vi "Read VI For Changes.vi"(8 "error in (no error)":errorcluster, 10 "Current VI Data":T1, 11 "VI Refnum":refnum<vi>) -> (0 "error out":errorcluster, 1 "ChangeInData?":bool, 2 "Updated VI Data":T1)   [LabVIEW 2014, in "SmartPalette.lvlib"]
uses:
  SmartPalette.lvlib
  Controls/VI - DataStorage.ctl
  Controls/GObjectDetail.ctl
  <vilib>/Utility/traverseref.llb/TRef TravTarget.ctl
  <vilib>/Utility/traverseref.llb/VI Scripting - Traverse.lvlib
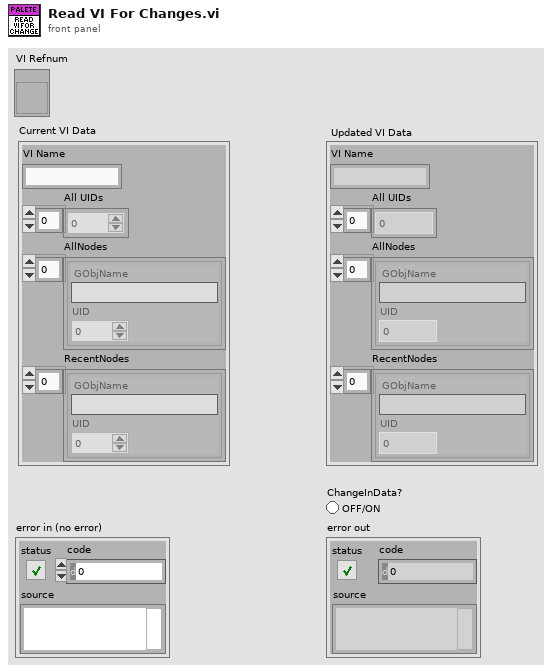
[diagram p1: front panel]
types:
  T1 = typedef "SmartPalette.lvlib/VI - DataStorage.ctl" = cluster{"VI Name":string, "All UIDs":i32[], "AllNodes":T2[], "RecentNodes":T2[]}
  T2 = typedef "SmartPalette.lvlib/GObjectDetail.ctl" = cluster{"GObjName":string, "UID":i32}
  T3 = typedef "TRef TravTarget.ctl" = enum16{"FP", "BD", "Other"}
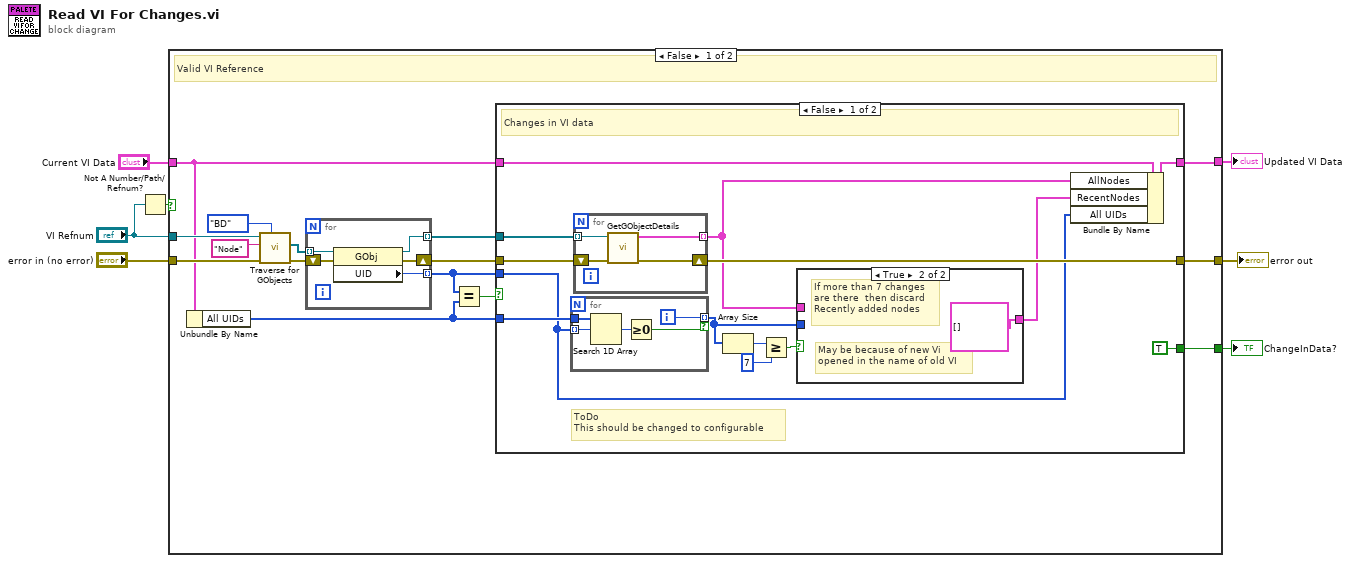
[diagram p0: block diagram]
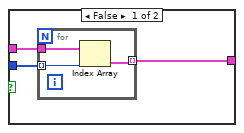
[diagram p2: hidden frame]
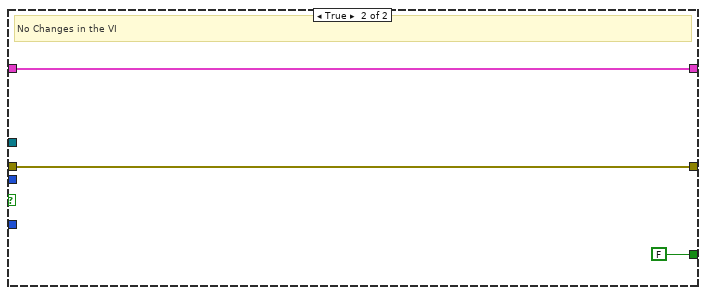
[diagram p3: hidden frame]
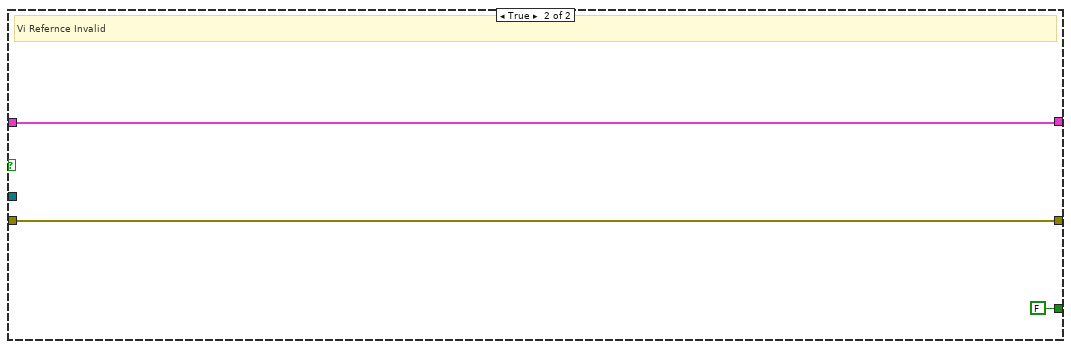
[diagram p4: hidden frame]
diagram:
  n1 = Not A Number/Path/Refnum?(number/path/refnum="VI Refnum") -> (NaN/Path/Refnum?=w4:bool)
  n2 = case shown="False" w4 {
    tunnel: "error in (no error)" -> [w22 w63]
    tunnel: [w15 w63] -> w6
    tunnel: "VI Refnum" -> [w20 _]
    tunnel: "Current VI Data" -> [w9 w62]
    tunnel: [w10 w62] -> w2
    tunnel: [w8 FALSE] -> w1
    frame False {
      # "Valid VI Reference"
      n3 = Unbundle By Name(w9) -> ("All UIDs"=w11:i32[])
      n4 = call <vilib>:"Traverse for GObjects.vi"("Traverse Target"=TRef_TravTarget."BD", "error in (no error)"=w22, "Class Name"="Node", "VI Refnum"=w20) -> ("error out"=w21:errorcluster, "References"=w17:refnum<vi>[])  [unwired: 4 in, 2 out]
      n5 = for {
        shift-right: [w59] -> w16
        shift-left: w21 -> [w60]
        tunnel: w17 -> [w58] mode=indexing
        tunnel: [w57] -> w12 mode=indexing
        tunnel: [w56] -> w13 mode=indexing
        n6 = property class="GObj"(reference=w58, error in=w60) -> (reference out=w56:refnum<vi>, error out=w59:errorcluster, "UID"=w57:i32)
      }
      n7 = Equal?(x=w12, y=w11) -> (x = y?=w14:bool)
      n8 = case shown="False" w14 {
        tunnel: w16 -> [w35 w55]
        tunnel: [w34 w55] -> w15
        tunnel: w13 -> [w33 _]
        tunnel: w12 -> [w24 _]
        tunnel: w11 -> [w36 _]
        tunnel: [w27 w54] -> w10
        tunnel: w9 -> [w28 w54]
        tunnel: [TRUE FALSE] -> w8
        frame False {
          # "ToDo\nThis should be changed to configurable"
          # "Changes in VI data"
          n9 = for {
            tunnel: w36 -> [w52]
            tunnel: w24 -> [w51] mode=indexing
            tunnel: [w50] -> w29 mode=indexing if=w49
            i -> [w50]
            n10 = Search 1D Array(1D array=w52, element=w51) -> (index of element=w48:i32)  [unwired: 1 in]
            n11 = Greater Or Equal To 0?(x=w48) -> (x >= 0?=w49:bool)
          }
          n12 = for {
            shift-right: [w46] -> w34
            shift-left: w35 -> [w47]
            tunnel: w33 -> [w45] mode=indexing
            tunnel: [w44] -> w26 mode=indexing
            n13 = call "GetGObjectDetails.vi"("error in (no error)"=w47, "GObject"=w45) -> ("error out"=w46:errorcluster, "output cluster"=w44:T2)  [unwired: 8 in]
          }
          n14 = Array Size(array=w29) -> (size(s)=w32:i32)
          n15 = Greater Or Equal?(x=w32, y=7) -> (x >= y?=w30:bool)
          n16 = case shown="True" w30 {
            tunnel: w26 -> [w39 _]
            tunnel: w29 -> [w38 _]
            tunnel: [w37 T2[] []] -> w25
            frame False {
              n17 = for {
                tunnel: w39 -> [w42]
                tunnel: w38 -> [w41] mode=indexing
                tunnel: [w40] -> w37 mode=indexing
                n18 = Index Array(array=w42, index=w41) -> (element=w40:T2)
              }
            }
            frame True {
              # "May be because of new Vi\nopened in the name of old VI"
              # "If more than 7 changes \nare there  then discard \nRecently added nodes"
            }
          }
          n19 = Bundle By Name(cluster=w28, "AllNodes"=w26, "RecentNodes"=w25, "All UIDs"=w24) -> (w27:T1)
        }
        frame True {
          # "No Changes in the VI"
        }
      }
    }
    frame True {
      # "Vi Refernce Invalid"
    }
  }
  "error out" <- w6
  "Updated VI Data" <- w2
  "ChangeInData?" <- w1
